vi "Get Cluster Data Size.vi"(8 "error in (no error)":errorcluster, 10 "Data String":u8[](array[numeric]), 11 "Type Descriptor":i16[](array[numeric])) -> (0 "error out":errorcluster, 2 "Data Size":i32)   [LabVIEW 2017, in "Composition.lvlib"]
doc: "Gets the data size of a cluster"
uses:
  Composition.lvlib
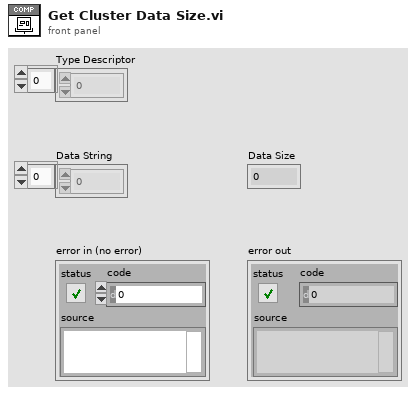
[diagram p1: front panel]
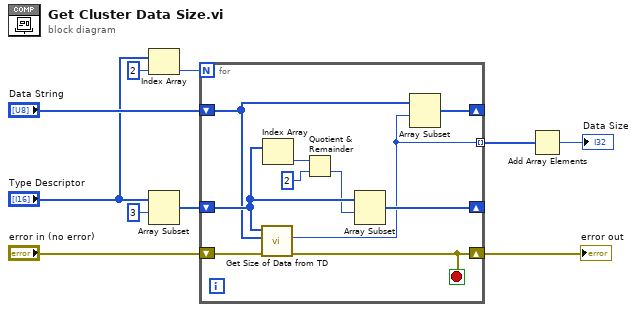
[diagram p0: block diagram]
diagram:
  n1 = Index Array(array="Type Descriptor", index=2) -> (element=w8:i16)
  n2 = Array Subset(array="Type Descriptor", index=3) -> (w6:i16[])  [unwired: 1 in]
  n3 = for {
    N: w8 -> [_]
    tunnel: [w13] -> w10 mode=indexing
    shift-right: [w19] -> _
    shift-left: w6 -> [w20]
    shift-right: [w14] -> _
    shift-left: "Data String" -> [w15]
    shift-right: [w11] -> w2
    shift-left: "error in (no error)" -> [w12]
    stop <- w11 stop-if-true
    n4 = call "Get Size of Data from TD.vi"("error in (no error)"=w12, "Data String"=w15, "Type Descriptor"=w20) -> ("error out"=w11:errorcluster, "Size of Data"=w13:i32)  [unwired: 7 in]
    n5 = Index Array(array=w20) -> (element=w17:i16)  [unwired: 1 in]
    n6 = Quotient & Remainder(x=w17, y=i16 2) -> (floor(x/y)=w18:i16)  [unwired: 1 out]
    n7 = Array Subset(array=w20, index=w18) -> (w19:i16[])  [unwired: 1 in]
    n8 = Array Subset(array=w15, index=w13) -> (w14:u8[])  [unwired: 1 in]
  }
  "error out" <- w2
  n9 = Add Array Elements(numeric array=w10) -> (sum=→"Data Size":i32)
